vi "Periodic Tasks.vi"(8 "error in":errorcluster) -> ()   [LabVIEW 2013]
doc: "This VI runs in parallel to other tasks. It can contain as many user-defined periodic loops as you need. These can carry out PID or other sorts of timed response."
uses:
  <vilib>/Platform/TimedLoop/XDataNode/timing_clust.ctl
  <vilib>/Platform/TimedLoop/XDataNode/nitl_modes.ctl
  <vilib>/Platform/TimedLoop/XDataNode/wakeup.ctl
  Robot Global Data.vi
  <vilib>/Rock Robotics/WPI/Solenoid/WPI_SolenoidSetEnum.vi
  <vilib>/Rock Robotics/WPI/Compressor/WPI_CompressorGetSetRefNum.vi
  <vilib>/platform/TimedLoop/XDataNode/XDataNode.xnode
  <vilib>/Platform/TimedLoop/XDataNode/XDNodeRunTimeDep.lvlib
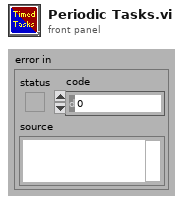
[diagram p1: front panel]
types:
  T1 = typedef "XDNodeRunTimeDep.lvlib/timing_clust.ctl" = cluster{"Expected End [f-1]":u64, "Actual End [f-1]":u64, "Finished Late? [f-1]":bool, "Expected End [i-1]":u64, "Actual End [i-1]":u64, "Finished Late? [i-1]":bool, "Expected Start [i]":u64, "Actual Start [i]":u64, "Expected Start [f]":u64, "Actual Start [f]":u64, "Source Name":string, "Structure Name":string, "Period":i64, "Deadline":i64, "Offset":i64, "Start":i64, "Priority":i32, "Timeout":i32, "Mode":T2, "Wakeup Reason":T3, "Error":errorcluster, "Source Type":string, "Secondary Source Type":string, "Global End Time":u64, "Global Start Time":u64, "Frame Duration":u64, "Iteration Duration":u64, "Assigned CPU":i32, "I/O Scan Engine Mode":u32}
  T2 = typedef "XDNodeRunTimeDep.lvlib/nitl_modes.ctl" = enum32{"No Change", "Process missed periods, maintain original phase", "Discard missed periods, maintain original phase", "Process missed periods, ignore original phase", "Discard missed periods, ignore original phase"}
  T3 = typedef "XDNodeRunTimeDep.lvlib/wakeup.ctl" = enum32{"Normal", "Aborted", "Asynchronous wakeup", "Timing source error", "Timed loop error", "Timeout"}
  T4 = typedef "WPI_SolenoidDevRef.ctl" = cluster{"DevStatus":errorcluster, "Solenoid Module":T5, "Forward Solenoid Channel":T6, "Reverse Solenoid Channel":T6}
  T5 = typedef "FPGA_TypedefSolenoidModule.ctl" = enum16{"Solenoid Module 1", "Solenoid Module 2"}
  T6 = typedef "WPI_SolenoidChannel.ctl" = enum8{"Solenoid 1", "Solenoid 2", "Solenoid 3", "Solenoid 4", "Solenoid 5", "Solenoid 6", "Solenoid 7", "Solenoid 8", "Invalid"}
  T7 = typedef "Shooter Manual Control.ctl" = cluster{"Command":T8, "Offset":dbl, "Trigger":bool, "Add":bool, "Release":bool, "Reset":bool, "Target Pressure":dbl, "Punch":bool, "AutoPunch":bool}
  T8 = typedef "Shooter Command.ctl" = enum16{"None", "Warmup", "Shoot", "Line Shoot", "Soft Shoot"}
  T9 = typedef "WPI_SolenoidValue.ctl" = enum16{"Off", "On", "Forward", "Reverse"}
  T10 = typedef "Shooter State.ctl" = enum16{"Wait", "Fill Piston", "Lift Halo", "Trigger", "Reset", "Soft Release", "Soft Unpin", "Soft Refill", "Soft Shoot"}
  T11 = typedef "WPI_CompressorDevRef.ctl" = cluster{"DevStatus":errorcluster, "DigitalInputDevRef":T12, "RelayDevRef":T15}
  T12 = typedef "WPI_DigitalInputDevRef.ctl" = cluster{"DevStatus":errorcluster, "DIO Channel":T13, "Digital Module":T14}
  T13 = typedef "FPGA_DIOChannel.ctl" = enum8{"DIO 1", "DIO 2", "DIO 3", "DIO 4", "DIO 5", "DIO 6", "DIO 7", "DIO 8", "DIO 9", "DIO 10", "DIO 11", "DIO 12", "DIO 13", "DIO 14", "Invalid"}
  T14 = typedef "FPGA_TypedefDigitalModule.ctl" = enum16{"Digital Module 1", "Digital Module 2"}
  T15 = typedef "WPI_RelayDevRef.ctl" = cluster{"DevStatus":errorcluster, "Relay Channel":T16, "Digital Module":T14, "Relay Direction":T17}
  T16 = typedef "FPGA_DIORelayChannel.ctl" = enum8{"Relay 1", "Relay 2", "Relay 3", "Relay 4", "Relay 5", "Relay 6", "Relay 7", "Relay 8", "Invalid"}
  T17 = typedef "WPI_RelayDirection.ctl" = enum16{"Both directions", "Forward only", "Reverse only"}
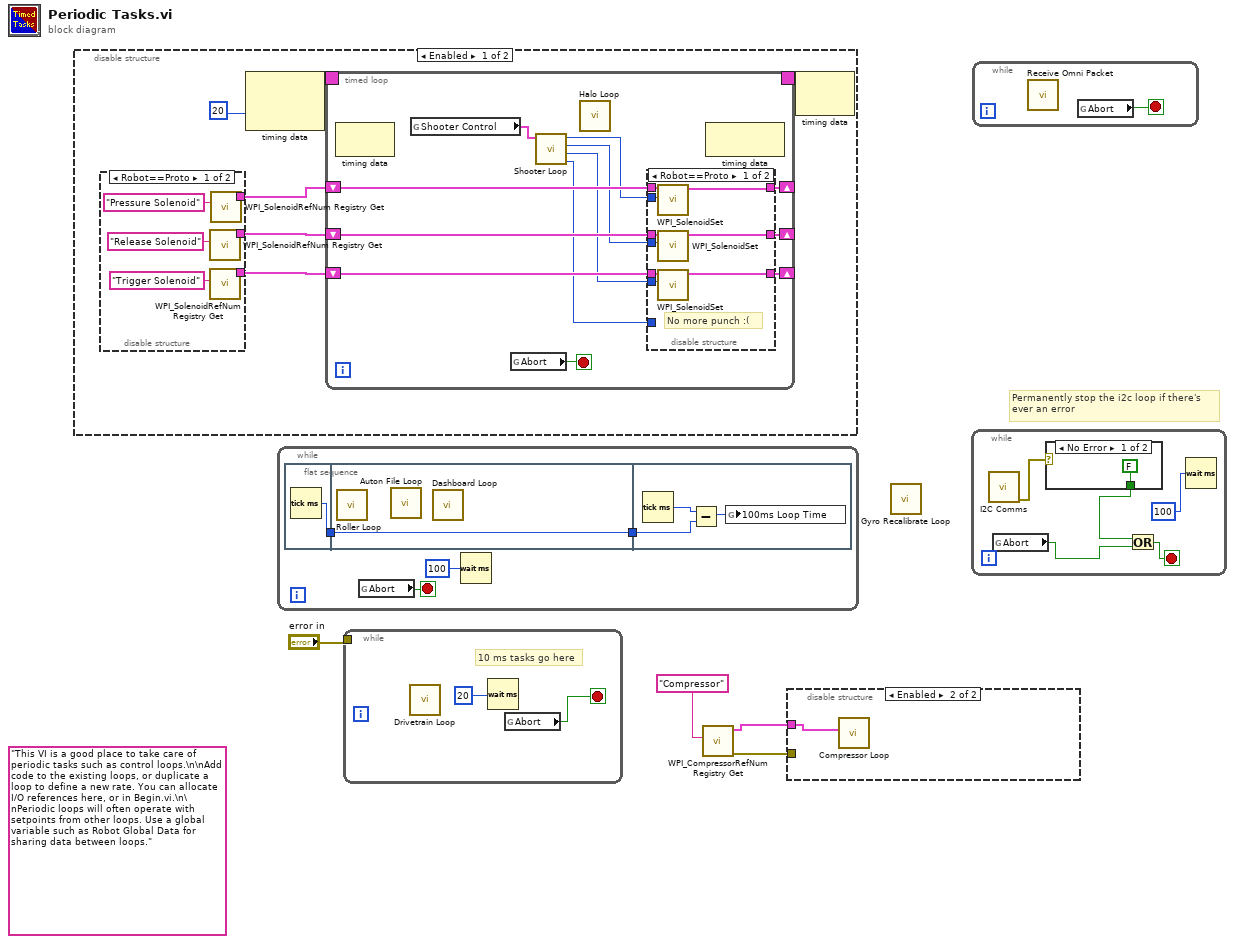
[diagram p0: block diagram]
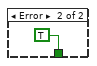
[diagram p2: hidden frame]
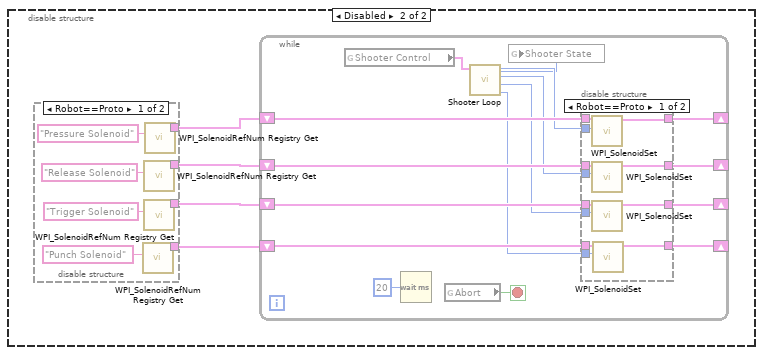
[diagram p5: hidden frame]
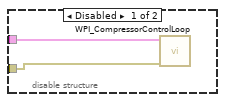
[diagram p8: hidden frame]
diagram:
  (unwired) "This VI is a good place to take care of periodic tasks such as control loops.\n\nAdd code to the existing loops, or duplicate a loop to define a new rate. You can allocate I/O references here, or in Begin.vi.\n\nPeriodic loops will often operate with setpoints from other loops. Use a global variable such as Robot Global Data for sharing data between loops."
  # "Permanently stop the i2c loop if there's\never an error"
  n1 = disable-structure shown="Enabled" {
    frame Enabled {
      n2 = disable-structure shown="Robot==Proto" {
        disable-tunnel: [w42 _] -> w10
        disable-tunnel: [w41 _] -> w9
        disable-tunnel: [w43 _] -> w8
        frame condition #0 (active) {
          n3 = call <vilib>:"WPI_SolenoidRefNum Registry Get.vi"("refnum name"="Release Solenoid") -> ("SolenoidDevRef"=w41:T4)  [unwired: 9 in, 1 out]
          n4 = call <vilib>:"WPI_SolenoidRefNum Registry Get.vi"("refnum name"="Trigger Solenoid") -> ("SolenoidDevRef"=w43:T4)  [unwired: 9 in, 1 out]
          n5 = call <vilib>:"WPI_SolenoidRefNum Registry Get.vi"("refnum name"="Pressure Solenoid") -> ("SolenoidDevRef"=w42:T4)  [unwired: 9 in, 1 out]
        }
        frame condition #1 {
        }
      }
      n6 = node-c288(u32 20 ("milliseconds to wait")) -> (w7:T1)  [unwired: 1 in]
      n7 = timed-loop {
        shift-right: [w19] -> _
        shift-left: w10 -> [w22]
        shift-right: [w18] -> _
        shift-left: w9 -> [w21]
        shift-right: [w17] -> _
        shift-left: w8 -> [w20]
        timing: w7 -> [_]
        timing-out: [_] -> w6
        stop <- w12 stop-if-true
        n8 = node-c288() -> ()  [unwired: 1 in, 1 out]
        n9 = global read "Robot Global Data.vi" "Shooter Control"() -> (w13:T7)
        n10 = global read "Robot Global Data.vi" "Abort"() -> (w12:bool)
        n11 = call "Shooter Loop.vi"("Shooter Control"=w13) -> ("Punch"=w11:T9, "Trigger"=w16:T9, "Release"=w15:T9, "Add"=w14:T9)  [unwired: 5 in, 2 out]
        n12 = call "Halo Loop.vi"() -> ()  [unwired: 12 in]
        n13 = disable-structure shown="Robot==Proto" {
          disable-tunnel: w22 -> [w25 _]
          disable-tunnel: w21 -> [w27 _]
          disable-tunnel: w20 -> [w32 _]
          disable-tunnel: [w33 _] -> w17
          disable-tunnel: [w28 _] -> w18
          disable-tunnel: [w26 _] -> w19
          disable-tunnel: w14 -> [w30 _]
          disable-tunnel: w15 -> [w29 _]
          disable-tunnel: w16 -> [w31 _]
          disable-tunnel: w11 -> [_ _]
          frame condition #0 (active) {
            # "No more punch :("
            n14 = call-poly <vilib>:"WPI_SolenoidSet.vi"("Value"=w30, "SolenoidDevRef"=w25) -> ("SolenoidDevRef"=w26:T4)  [unwired: 8 in, 1 out]
            n15 = call-poly <vilib>:"WPI_SolenoidSet.vi"("Value"=w29, "SolenoidDevRef"=w27) -> ("SolenoidDevRef"=w28:T4)  [unwired: 8 in, 1 out]
            n16 = call-poly <vilib>:"WPI_SolenoidSet.vi"("Value"=w31, "SolenoidDevRef"=w32) -> ("SolenoidDevRef"=w33:T4)  [unwired: 8 in, 1 out]
          }
          frame condition #1 {
          }
        }
        n17 = node-c288() -> ()  [unwired: 1 in, 1 out]
      }
      n18 = node-c288(w6) -> ()  [unwired: 1 out]
    }
    frame Disabled {
      n19 = disable-structure shown="Robot==Proto" {
        disable-tunnel: [w54 _] -> w47
        disable-tunnel: [w53 _] -> w46
        disable-tunnel: [w55 _] -> w45
        disable-tunnel: [w49 _] -> w44
        frame condition #0 (active) {
          n20 = call <vilib>:"WPI_SolenoidRefNum Registry Get.vi"("refnum name"="Punch Solenoid") -> ("SolenoidDevRef"=w49:T4)  [unwired: 9 in, 1 out]
          n21 = call <vilib>:"WPI_SolenoidRefNum Registry Get.vi"("refnum name"="Release Solenoid") -> ("SolenoidDevRef"=w53:T4)  [unwired: 9 in, 1 out]
          n22 = call <vilib>:"WPI_SolenoidRefNum Registry Get.vi"("refnum name"="Trigger Solenoid") -> ("SolenoidDevRef"=w55:T4)  [unwired: 9 in, 1 out]
          n23 = call <vilib>:"WPI_SolenoidRefNum Registry Get.vi"("refnum name"="Pressure Solenoid") -> ("SolenoidDevRef"=w54:T4)  [unwired: 9 in, 1 out]
        }
        frame condition #1 {
        }
      }
      n24 = while {
        shift-right: [w68] -> _
        shift-left: w47 -> [w71]
        shift-right: [w67] -> _
        shift-left: w46 -> [w70]
        shift-right: [w66] -> _
        shift-left: w45 -> [w69]
        shift-right: [w58] -> _
        shift-left: w44 -> [w57]
        stop <- w59 stop-if-true
        n25 = global read "Robot Global Data.vi" "Shooter Control"() -> (w60:T7)
        n26 = Wait (ms)(milliseconds to wait=u32 20) -> ()  [unwired: 1 out]
        n27 = global read "Robot Global Data.vi" "Abort"() -> (w59:bool)
        n28 = call "Shooter Loop.vi"("Shooter Control"=w60) -> ("Punch"=w56:T9, "Trigger"=w64:T9, "Release"=w63:T9, "Add"=w62:T9, "State"=w61:T10)  [unwired: 5 in, 1 out]
        n29 = global write "Robot Global Data.vi" "Shooter State"(w61) -> ()
        n30 = disable-structure shown="Robot==Proto" {
          disable-tunnel: w71 -> [w75 _]
          disable-tunnel: w70 -> [w77 _]
          disable-tunnel: w69 -> [w82 _]
          disable-tunnel: [w83 _] -> w66
          disable-tunnel: [w78 _] -> w67
          disable-tunnel: [w76 _] -> w68
          disable-tunnel: w62 -> [w80 _]
          disable-tunnel: w63 -> [w79 _]
          disable-tunnel: w64 -> [w81 _]
          disable-tunnel: [w74 _] -> w58
          disable-tunnel: w57 -> [w73 _]
          disable-tunnel: w56 -> [w72 _]
          frame condition #0 (active) {
            n31 = call-poly <vilib>:"WPI_SolenoidSet.vi"("Value"=w80, "SolenoidDevRef"=w75) -> ("SolenoidDevRef"=w76:T4)  [unwired: 8 in, 1 out]
            n32 = call-poly <vilib>:"WPI_SolenoidSet.vi"("Value"=w79, "SolenoidDevRef"=w77) -> ("SolenoidDevRef"=w78:T4)  [unwired: 8 in, 1 out]
            n33 = call-poly <vilib>:"WPI_SolenoidSet.vi"("Value"=w81, "SolenoidDevRef"=w82) -> ("SolenoidDevRef"=w83:T4)  [unwired: 8 in, 1 out]
            n34 = call-poly <vilib>:"WPI_SolenoidSet.vi"("Value"=w72, "SolenoidDevRef"=w73) -> ("SolenoidDevRef"=w74:T4)  [unwired: 8 in, 1 out]
          }
          frame condition #1 {
          }
        }
      }
    }
  }
  n35 = while {
    stop <- w86 stop-if-true
    n36 = flat-sequence {
      tunnel: [w88] -> w85
      tunnel: w85 -> [w89]
      tunnel: [w89] -> w84
      tunnel: w84 -> [w91]
      frame #0 {
        n37 = Tick Count (ms)() -> (millisecond timer value=w88:u32)
      }
      frame #1 {
        n38 = call "Roller Loop.vi"() -> ()  [unwired: 12 in]
        n39 = call "Auton File Loop.vi"() -> ()  [unwired: 12 in]
        n40 = call "Dashboard Loop.vi"() -> ()  [unwired: 12 in]
      }
      frame #2 {
        n41 = Tick Count (ms)() -> (millisecond timer value=w92:u32)
        n42 = Subtract(x=w92, y=w91) -> (x-y=w90:u32)
        n43 = global write "Robot Global Data.vi" "100ms Loop Time"(w90) -> ()
      }
    }
    n44 = global read "Robot Global Data.vi" "Abort"() -> (w86:bool)
    n45 = Wait (ms)(milliseconds to wait=u32 100 ("millisecond multiple")) -> ()  [unwired: 1 out]
  }
  n46 = while {
    tunnel: "error in" -> [_]
    stop <- w93 stop-if-true
    # "10 ms tasks go here"
    n47 = call "Drivetrain Loop.vi"() -> ()  [unwired: 12 in]
    n48 = Wait (ms)(milliseconds to wait=u32 20) -> ()  [unwired: 1 out]
    n49 = global read "Robot Global Data.vi" "Abort"() -> (w93:bool)
  }
  n50 = call <vilib>:"WPI_CompressorRefNum Registry Get.vi"("refnum name"="Compressor") -> ("error out"=w2:errorcluster, "CompressorDevRef"=w1:T11)  [unwired: 9 in]
  n51 = disable-structure shown="Enabled" {
    disable-tunnel: w1 -> [w96 w97]
    disable-tunnel: w2 -> [w95 _]
    frame Disabled {
      n52 = call <vilib>:"WPI_CompressorControlLoop.vi"("error in (no error)"=w95, "CompressorDevRef"=w96) -> ()  [unwired: 10 in]
    }
    frame Enabled {
      n53 = call "Compressor Loop.vi"("CompressorDevRef"=w97) -> ()  [unwired: 11 in]
    }
  }
  n54 = call "Gyro Recalibrate Loop.vi"() -> ()  [unwired: 12 in]
  n55 = while {
    stop <- w99 stop-if-true
    n56 = call "I2C Comms.vi"() -> ("error out"=w102:errorcluster)  [unwired: 10 in, 1 out]
    n57 = global read "Robot Global Data.vi" "Abort"() -> (w101:bool)
    n58 = case shown="No Error" w102 {
      tunnel: [FALSE TRUE] -> w100
      frame No Error {
      }
      frame Error {
      }
    }
    n59 = Or(x=w100, y=w101) -> (x .or. y?=w99:bool)
    n60 = Wait (ms)(milliseconds to wait=u32 100 ("millisecond multiple")) -> ()  [unwired: 1 out]
  }
  n61 = while {
    stop <- w105 stop-if-true
    n62 = call "Receive Omni Packet.vi"() -> ()  [unwired: 12 in]
    n63 = global read "Robot Global Data.vi" "Abort"() -> (w105:bool)
  }
